vi "Get Control Screen Position.vi"(11 "Control in":refnum<vi>) -> (3 "Bounds Out":T1)   [LabVIEW 2020]
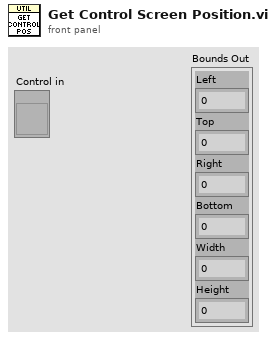
[diagram p1: front panel]
types:
  T1 = cluster{"Left":i16, "Top":i16, "Right":i16, "Bottom":i16, "Width":i16, "Height":i16}
  T2 = typedef "LVPositionTypeDef.ctl" = cluster{"Left":i32, "Top":i32}
  T3 = typedef "LVBoundsTypeDef.ctl" = cluster{"Width":u32, "Height":u32}
  T4 = typedef "LVRectTypeDef.ctl" = cluster{"Left":i16, "Top":i16, "Right":i16, "Bottom":i16}
  T5 = typedef "LVPointTypeDef.ctl" = cluster{"Horizontal":i16, "Vertical":i16}
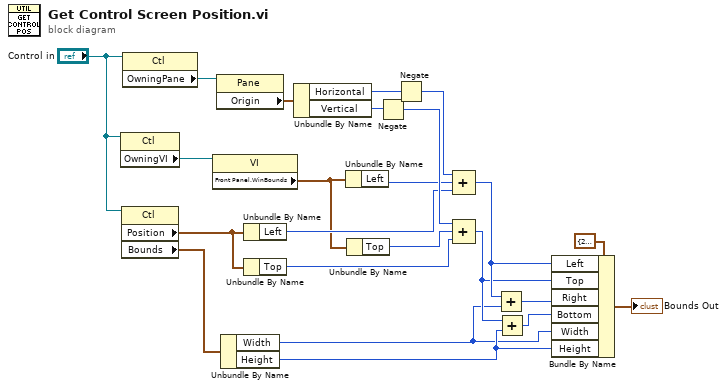
[diagram p0: block diagram]
diagram:
  n1 = property class="Ctl"(reference="Control in") -> ("OwningVI"=w1:refnum<vi>)  [unwired: 1 in, 2 out]
  n2 = property class="Ctl"(reference="Control in") -> ("Position"=w16:T2, "Bounds"=w10:T3)  [unwired: 1 in, 2 out]
  n3 = property class="Ctl"(reference="Control in") -> ("OwningPane"=w18:refnum<vi>)  [unwired: 1 in, 2 out]
  n4 = property class="VI"(reference=w1) -> ("Front Panel.WinBounds"=w2:T4)  [unwired: 1 in, 2 out]
  n5 = property class="Pane"(reference=w18) -> ("Origin"=w19:T5)  [unwired: 1 in, 2 out]
  n6 = Unbundle By Name(w10) -> ("Width"=w4:u32, "Height"=w5:u32)
  n7 = Unbundle By Name(w16) -> ("Left"=w13:i32)
  n8 = Unbundle By Name(w16) -> ("Top"=w15:i32)
  n9 = Unbundle By Name(w19) -> ("Horizontal"=w20:i16, "Vertical"=w21:i16)
  n10 = Unbundle By Name(w2) -> ("Left"=w12:i16)
  n11 = Unbundle By Name(w2) -> ("Top"=w14:i16)
  n12 = Negate(x=w21) -> (-x=w23:i16)
  n13 = Negate(x=w20) -> (-x=w22:i16)
  n14 = Compound Arithmetic op=ADD(w22, w12, w13) -> (w8:i32)
  n15 = Compound Arithmetic op=ADD(w23, w14, w15) -> (w7:i32)
  n16 = Add(x=w8, y=w4) -> (x+y=w9:u32)
  n17 = Add(x=w7, y=w5) -> (x+y=w6:u32)
  n18 = Bundle By Name(cluster=T1 {"Left"=2174, "Top"=366, "Right"=2650, "Bottom"=811, "Width"=476, "Height"=445} ("Bounds Out"), "Left"=w8, "Top"=w7, "Right"=w9, "Bottom"=w6, "Width"=w4, "Height"=w5) -> (→"Bounds Out":T1)
